vi "binaryOutputs.vi"(8 "TimedOut":bool, 11 "OutputPortU8":u8) -> ()   [LabVIEW 2018]
doc: "This vi contains connections to the digital outputs. The motor power output is set to power off if the Timeout input is true."
uses:
  <vilib>/rvi/eio/common/nirviEmuTemplateMethod_errors.vi
  <vilib>/eio/EIONode/EIONode.xnode
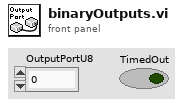
[diagram p1: front panel]
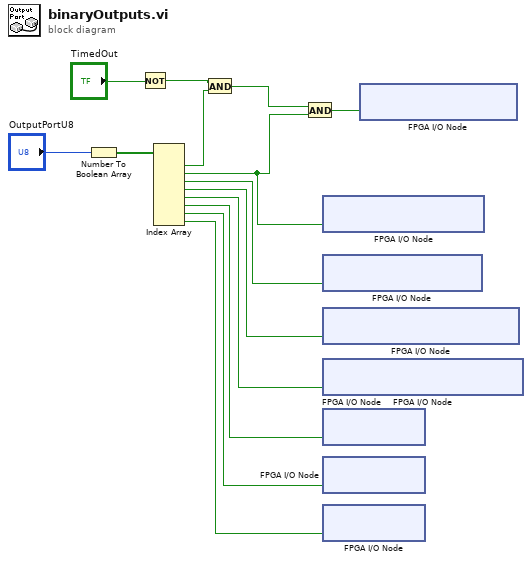
[diagram p0: block diagram]
diagram:
  n1 = Number To Boolean Array(number="OutputPortU8") -> (Boolean array=w13:bool[])
  n2 = Not(x="TimedOut") -> (.not. x?=w5:bool)
  n3 = Index Array(array=w13) -> (element #1=w6:bool, element #2=w1:bool, element #3=w7:bool, element #4=w8:bool, element #5=w9:bool, element #6=w10:bool, element #7=w11:bool, element #8=w12:bool)  [unwired: 8 in]
  n4 = And(x=w5, y=w6) -> (x .and. y?=w2:bool)
  n5 = And(x=w2, y=w1) -> (x .and. y?=w3:bool)
  n6 = xnode "FPGA I/O Node"("ILC_Comm_Power_On"=w1) -> ()  [unwired: 1 in, 1 out]
  n7 = xnode "FPGA I/O Node"("cRIO_Interlock_Enable"=w7) -> ()  [unwired: 1 in, 1 out]
  n8 = xnode "FPGA I/O Node"("Reset_Motor_Power_Breakers"=w8) -> ()  [unwired: 1 in, 1 out]
  n9 = xnode "FPGA I/O Node"("Reset_Comm_Power_Breakers"=w9) -> ()  [unwired: 1 in, 1 out]
  n10 = xnode "FPGA I/O Node"("Mod4/CH5"=w10) -> ()  [unwired: 1 in, 1 out]
  n11 = xnode "FPGA I/O Node"("Mod4/CH6"=w11) -> ()  [unwired: 1 in, 1 out]
  n12 = xnode "FPGA I/O Node"("Mod4/CH7"=w12) -> ()  [unwired: 1 in, 1 out]
  n13 = xnode "FPGA I/O Node"("ILC_Motor_Power_On"=w3) -> ()  [unwired: 1 in, 1 out]
